vi "1553 Address Based Handles to Execution Unit Address Handles.vi"(8 "error in":errorcluster, 11 "1553 address based channel handles":T1 {"acyclic frame trigger handles"."handle" format="%.0x"; "start stop handles"."stop handle" format="%.0x"; "start stop handles"."start handle" format="%.0x"}) -> (0 "error out":errorcluster, 3 "address based channels":T4[](array[typedef]) format="%.0x")   [LabVIEW 2020, in "AIM MIL-STD-1553 Engine.lvlib" / "Implementation.lvlib" / "Tx Acyclic Execution Unit.lvclass"]
uses:
  Tx Acyclic Execution Unit.lvclass
  <vilib>/NI VeriStand/Custom Device API/Custom Device Item Ref.ctl
  <vilib>/NI VeriStand/Custom Device API/Custom Device API.lvlib
  Shared/Address.ctl
  Start Stop Channel Handles.ctl
  1553 Address Based Handles.ctl
  Acyclic Frame Trigger Handle.ctl
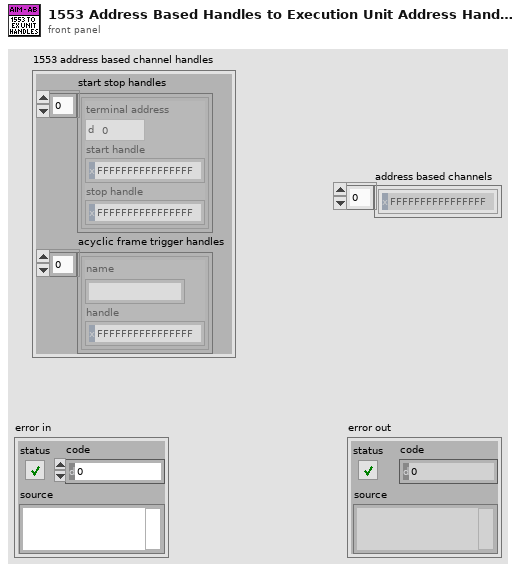
[diagram p1: front panel]
types:
  T1 = typedef "AIM MIL-STD-1553 Engine.lvlib/Implementation.lvlib/Tx Acyclic Execution Unit.lvclass/1553 Address Based Handles.ctl" = cluster{"start stop handles":T2[], "acyclic frame trigger handles":T5[]}
  T2 = typedef "AIM MIL-STD-1553 Engine.lvlib/Implementation.lvlib/Tx Acyclic Execution Unit.lvclass/Start Stop Channel Handles.ctl" = cluster{"terminal address":T3, "start handle":T4, "stop handle":T4}
  T3 = typedef "Address.ctl" = u16
  T4 = typedef "Custom Device API.lvlib/Custom Device Item Ref.ctl" = u64
  T5 = typedef "AIM MIL-STD-1553 Engine.lvlib/Implementation.lvlib/Tx Acyclic Execution Unit.lvclass/Acyclic Frame Trigger Handle.ctl" = cluster{"name":string, "handle":T4}
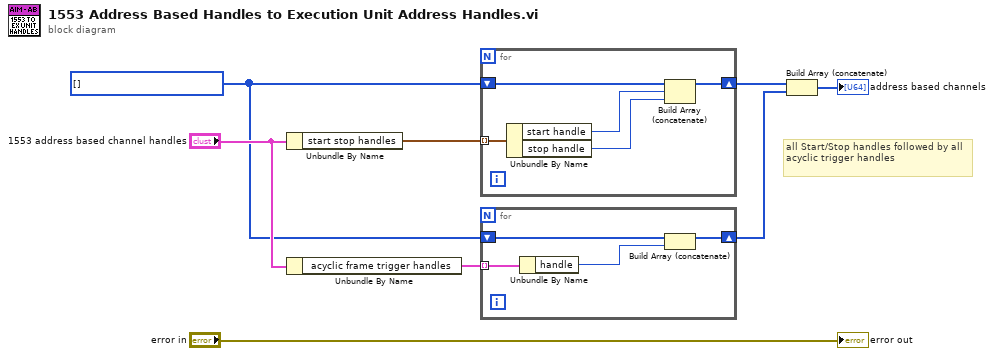
[diagram p0: block diagram]
diagram:
  w6 = T4[] [] ("Incoming Channels")
  # "all Start/Stop handles followed by all acyclic trigger handles"
  n1 = Unbundle By Name("1553 address based channel handles") -> ("start stop handles"=w2:T2[])
  n2 = Unbundle By Name("1553 address based channel handles") -> ("acyclic frame trigger handles"=w1:T5[])
  n3 = for {
    shift-right: [w12] -> w5
    shift-left: w6 -> [w13]
    tunnel: w2 -> [w11] mode=indexing
    n4 = Unbundle By Name(w11) -> ("start handle"=w10:T4, "stop handle"=w9:T4)
    n5 = Build Array (concatenate)(w13, w10, w9) -> (w12:T4[])
  }
  n6 = for {
    shift-right: [w16] -> w3
    shift-left: w6 -> [w17]
    tunnel: w1 -> [w15] mode=indexing
    n7 = Unbundle By Name(w15) -> ("handle"=w14:T4)
    n8 = Build Array (concatenate)(w17, w14) -> (w16:T4[])
  }
  n9 = Build Array (concatenate)(w5, w3) -> (→"address based channels":T4[])
  "error out" <- "error in"
